vi "SubDiameter.vi"(7 "Calibration (1 pixel = ?um)":dbl=1.45, 8 "error in (no error)":errorcluster, 9 "Bot Wall":T1 {"Y" format="%.2f"; "X" format="%.2f"}, 10 "Top wall":T1 {"Y" format="%.2f"; "X" format="%.2f"}, 11 "AVI Path":path) -> (0 "error out":errorcluster, 1 "Y Mid":sgl[](array[numeric]), 2 "X Mid":sgl[](array[numeric]), 3 "Diameter":dbl[](array[numeric]))   [LabVIEW 2017]
uses:
  <vilib>/vision/NI_Vision_Development_Module.lvlib
panel:
  out "Vessel Diameter":dbl[](graph)
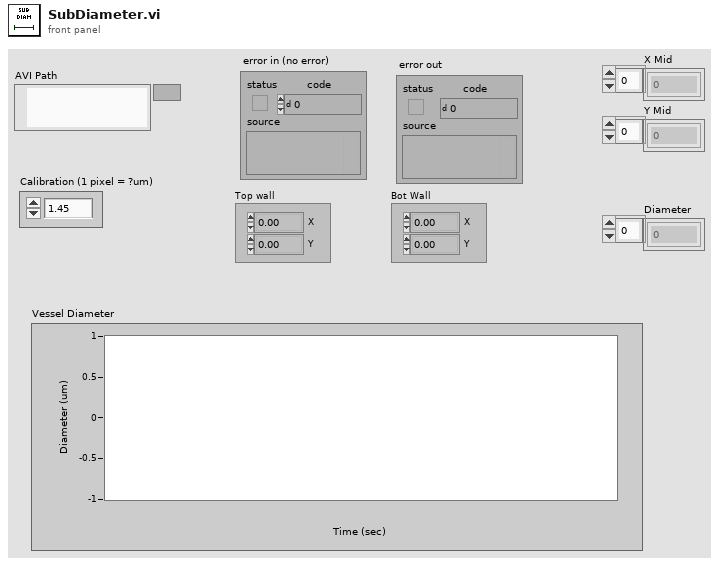
[diagram p1: front panel]
types:
  T1 = typedef "IMAQ Point" = cluster{"X":sgl, "Y":sgl}
  T2 = typedef "Image Type" = u32
  T3 = typedef "IMAQ AVI2 Refnum.ctl" = refnum<k20>
  T4 = cluster{"Width":u32, "Height":u32, "Frames Per Second":u32, "Codec":string, "Has Data":bool}
  T5 = typedef "IMAQ Image.ctl" = refnum<image>
  T6 = typedef "ROI Descriptor" = cluster{"Global Rectangle":i32[], "Contours":cluster{"ID":enum32{"External", "Internal"}, "Type":u32, "Coordinates":i32[]}[]}
  T7 = cluster{"Position":cluster{"x":sgl, "y":sgl}, "Angle":sgl, "Scale":sgl, "Score":sgl, "Bounding Box":cluster{"x":sgl, "y":sgl}[]}[]
  T8 = cluster{"Position":cluster{"x":sgl, "y":sgl}, "Position":cluster{"x":sgl, "y":sgl}}
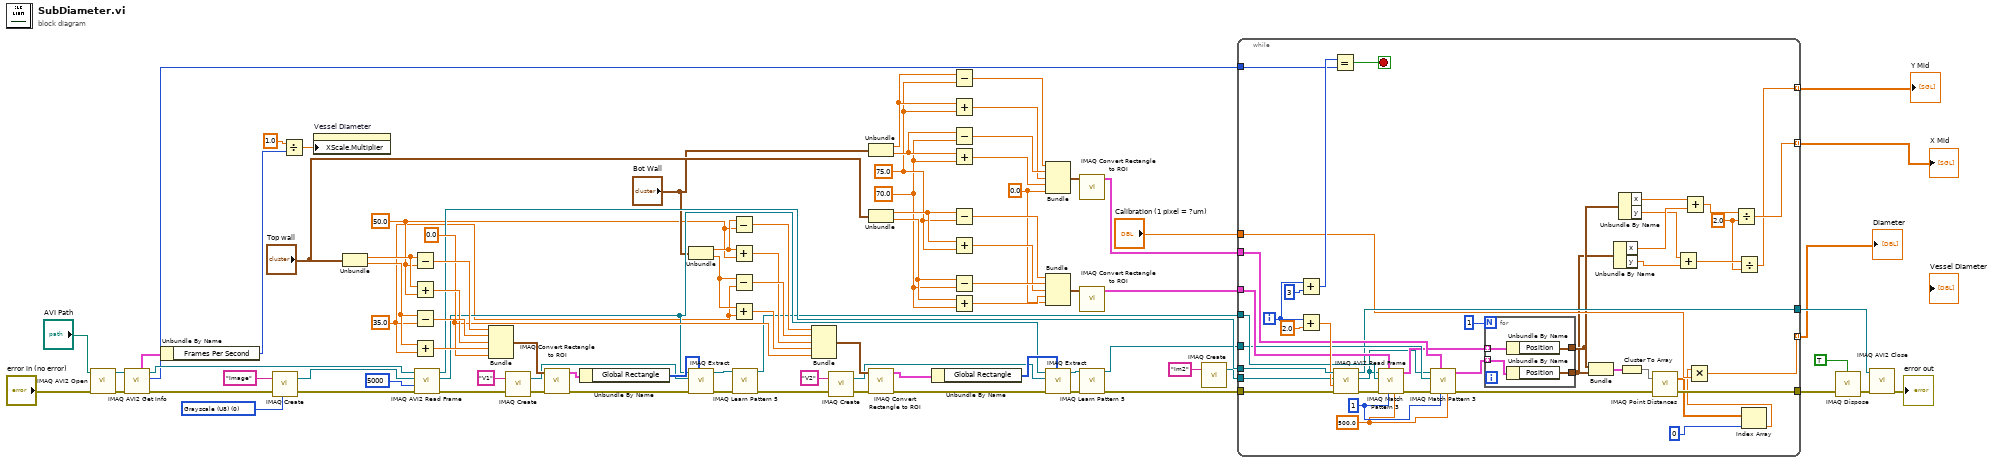
[diagram p0: block diagram]
diagram:
  w5 = 70.0 ("Search region offset (y)")
  w6 = 75.0 ("Search region offset (x)")
  w7 = 35.0 ("Reference offset (y)")
  w8 = 50.0 ("Reference offset (x)")
  w33 = 0.0
  w65 = 0.0
  w82 = T2 0 items=["Grayscale (U8)", "Grayscale (I16)", "Grayscale (SGL)", "Complex (CSG)", "RGB (U32)", "HSL (U32)", "RGB (U64)", "Grayscale (U16)"] ("Image Type")
  n1 = call "IMAQ AVI2 Open"("error in (no error)"="error in (no error)", "AVI File Path"="AVI Path") -> ("error out"=w88:errorcluster, "AVI Refnum"=w87:T3)  [unwired: 8 in]
  n2 = call "IMAQ AVI2 Get Info"("error in (no error)"=w88, "AVI Refnum"=w87) -> ("error out"=w85:errorcluster, "Number of Frames"=w46:u32, "AVI Refnum (duplicate)"=w80:T3, "Frame Data"=w23:T4)  [unwired: 5 in, 1 out]
  n3 = Unbundle By Name(w23) -> ("Frames Per Second"=w21:u32)
  n4 = call "IMAQ Create"("Image Name"="Image", "Image Type"=w82, "error in (no error)"=w85) -> ("New Image"=w84:T5, "error out"=w83:errorcluster)  [unwired: 2 in]
  n5 = Divide(x=1.0, y=w21) -> (x/y=w20:dbl)
  n6 = property on="Vessel Diameter" class="WFChart (strict)"("XScale.Multiplier"=w20) -> ()  [unwired: 2 in, 2 out]
  n7 = Unbundle("Top wall") -> ("X"=w79:sgl, "Y"=w78:sgl)
  n8 = Subtract(x=w79, y=w8) -> (x-y=w75:dbl)
  n9 = Add(x=w79, y=w8) -> (x+y=w73:dbl)
  n10 = Subtract(x=w78, y=w7) -> (x-y=w74:dbl)
  n11 = Add(x=w78, y=w7) -> (x+y=w72:dbl)
  n12 = call "IMAQ AVI2 Read Frame"("error in (no error)"=w83, "Frame Number"=u32 5000, "Image"=w84, "AVI Refnum"=w80) -> ("error out"=w11:errorcluster, "Image Out"=w52:T5, "AVI Refnum (duplicate)"=w47:T3)  [unwired: 5 in]
  n13 = Bundle(w75, w74, w73, w72, w65) -> (w71:cluster{dbl, dbl, dbl, dbl, dbl})  [unwired: 1 in]
  n14 = call "IMAQ Create"("Image Name"="V1", "error in (no error)"=w11) -> ("New Image"=w54:T5, "error out"=w62:errorcluster)  [unwired: 3 in]
  n15 = call "IMAQ Convert Rectangle to ROI"("error in (no error)"=w62, "Rectangle"=w71) -> ("error out"=w55:errorcluster, "ROI Descriptor"=w58:T6)  [unwired: 7 in]
  n16 = Unbundle By Name(w58) -> ("Global Rectangle"=w57:i32[])
  n17 = Unbundle("Bot Wall") -> ("X"=w77:sgl, "Y"=w76:sgl)
  n18 = call "IMAQ Extract"("Optional Rectangle"=w57, "error in (no error)"=w55, "Image Dst"=w54, "Image Src"=w52) -> ("error out"=w51:errorcluster, "Image Dst Out"=w50:T5)  [unwired: 6 in]
  n19 = Subtract(x=w77, y=w8) -> (x-y=w69:dbl)
  n20 = Add(x=w77, y=w8) -> (x+y=w67:dbl)
  n21 = Subtract(x=w76, y=w7) -> (x-y=w68:dbl)
  n22 = Add(x=w76, y=w7) -> (x+y=w66:dbl)
  n23 = call "IMAQ Learn Pattern 5"("Image"=w50, "error in (no error)"=w51) -> ("Template Image Out"=w30:T5, "error out"=w28:errorcluster)  [unwired: 11 in, 1 out]
  n24 = Bundle(w69, w68, w67, w66, w65) -> (w70:cluster{dbl, dbl, dbl, dbl, dbl})  [unwired: 1 in]
  n25 = call "IMAQ Create"("Image Name"="V2", "error in (no error)"=w28) -> ("New Image"=w53:T5, "error out"=w61:errorcluster)  [unwired: 3 in]
  n26 = Unbundle("Bot Wall") -> ("X"=w35:sgl, "Y"=w34:sgl)
  n27 = Unbundle("Top wall") -> ("X"=w41:sgl, "Y"=w40:sgl)
  n28 = call "IMAQ Convert Rectangle to ROI"("error in (no error)"=w61, "Rectangle"=w70) -> ("error out"=w56:errorcluster, "ROI Descriptor"=w60:T6)  [unwired: 7 in]
  n29 = Unbundle By Name(w60) -> ("Global Rectangle"=w59:i32[])
  n30 = Subtract(x=w35, y=w6) -> (x-y=w39:dbl)
  n31 = Add(x=w35, y=w6) -> (x+y=w37:dbl)
  n32 = Subtract(x=w34, y=w5) -> (x-y=w38:dbl)
  n33 = Add(x=w34, y=w5) -> (x+y=w36:dbl)
  n34 = Subtract(x=w41, y=w6) -> (x-y=w45:dbl)
  n35 = Add(x=w41, y=w6) -> (x+y=w43:dbl)
  n36 = Subtract(x=w40, y=w5) -> (x-y=w44:dbl)
  n37 = Add(x=w40, y=w5) -> (x+y=w42:dbl)
  n38 = Bundle(w39, w38, w37, w36, w33) -> (w25:cluster{dbl, dbl, dbl, dbl, dbl})  [unwired: 1 in]
  n39 = Bundle(w45, w44, w43, w42, w33) -> (w26:cluster{dbl, dbl, dbl, dbl, dbl})  [unwired: 1 in]
  n40 = call "IMAQ Extract"("Optional Rectangle"=w59, "error in (no error)"=w56, "Image Dst"=w53, "Image Src"=w52) -> ("error out"=w49:errorcluster, "Image Dst Out"=w48:T5)  [unwired: 6 in]
  n41 = call "IMAQ Convert Rectangle to ROI"("Rectangle"=w25) -> ("ROI Descriptor"=w31:T6)  [unwired: 8 in, 1 out]
  n42 = call "IMAQ Convert Rectangle to ROI"("Rectangle"=w26) -> ("ROI Descriptor"=w32:T6)  [unwired: 8 in, 1 out]
  n43 = call "IMAQ Learn Pattern 5"("Image"=w48, "error in (no error)"=w49) -> ("Template Image Out"=w29:T5, "error out"=w27:errorcluster)  [unwired: 11 in, 1 out]
  n44 = call "IMAQ Create"("Image Name"="Im2") -> ("New Image"=w18:T5)  [unwired: 4 in, 1 out]
  n45 = while {
    tunnel: w47 -> [w131]
    tunnel: w46 -> [w125]
    tunnel: w32 -> [w123]
    tunnel: w31 -> [w122]
    tunnel: w30 -> [w119]
    tunnel: w29 -> [w118]
    tunnel: w27 -> [w117]
    tunnel: [w109] -> w24
    tunnel: w18 -> [w107]
    tunnel: [w105] -> w15
    tunnel: "Calibration (1 pixel = ?um)" -> [w104]
    tunnel: [w103] -> w1 mode=indexing
    tunnel: [w93] -> w3 mode=indexing
    tunnel: [w92] -> w2 mode=indexing
    i -> [w128]
    stop <- w124 stop-if-true
    w94 = sgl 2.0 ("y")
    w108 = sgl 500.0 ("Minimum Match Score")
    w116 = 1 ("Number of Matches Requested")
    n46 = Add(x=w128, y=3) -> (x+y=w126:i32)
    n47 = Add(x=w128, y=2.0) -> (x+y=w129:dbl)
    n48 = Equal?(x=w126, y=w125) -> (x = y?=w124:bool)
    n49 = call "IMAQ AVI2 Read Frame"("error in (no error)"=w117, "Frame Number"=w129, "Image"=w107, "AVI Refnum"=w131) -> ("error out"=w121:errorcluster, "Image Out"=w112:T5, "AVI Refnum (duplicate)"=w109:T3)  [unwired: 5 in]
    n50 = call "IMAQ Match Pattern 3"("Minimum Match Score"=w108, "Number of Matches Requested"=w116, "ROI Descriptor"=w123, "error in (no error)"=w121, "Template Image"=w119, "Image"=w112) -> ("error out"=w120:errorcluster, "Matches"=w114:T7)  [unwired: 3 in, 1 out]
    n51 = call "IMAQ Match Pattern 3"("Minimum Match Score"=w108, "Number of Matches Requested"=w116, "ROI Descriptor"=w122, "error in (no error)"=w120, "Template Image"=w118, "Image"=w112) -> ("error out"=w106:errorcluster, "Matches"=w113:T7)  [unwired: 3 in, 1 out]
    n52 = for {
      N: 1 -> [_]
      tunnel: w114 -> [w135] mode=indexing
      tunnel: w113 -> [w134] mode=indexing
      tunnel: [w133] -> w102
      tunnel: [w132] -> w101
      n53 = Unbundle By Name(w135) -> ("Position"=w133:cluster{"x":sgl, "y":sgl})
      n54 = Unbundle By Name(w134) -> ("Position"=w132:cluster{"x":sgl, "y":sgl})
    }
    n55 = Bundle("Position"=w102, "Position"=w101) -> (w110:T8)  [unwired: 1 in]
    n56 = Unbundle By Name(w101) -> ("x"=w99:sgl, "y"=w96:sgl)
    n57 = Unbundle By Name(w102) -> ("x"=w100:sgl, "y"=w97:sgl)
    n58 = Cluster To Array(cluster=w110) -> (array=w111:cluster{"x":sgl, "y":sgl}[])
    n59 = call "IMAQ Point Distances"("Points"=w111, "error in (no error)"=w106) -> ("Distances"=w91:sgl[], "error out"=w105:errorcluster)  [unwired: 3 in]
    n60 = Add(x=w97, y=w96) -> (x+y=w95:sgl)
    n61 = Add(x=w100, y=w99) -> (x+y=w98:sgl)
    n62 = Divide(x=w98, y=w94) -> (x/y=w93:sgl)
    n63 = Divide(x=w95, y=w94) -> (x/y=w92:sgl)
    n64 = Index Array(array=w91, index=0 ("index (row)")) -> (element=w89:sgl)
    n65 = Multiply(x=w89, y=w104) -> (x*y=w103:dbl)
  }
  "Diameter" <- w1
  "X Mid" <- w3
  "Y Mid" <- w2
  n66 = call "IMAQ Dispose"("All Images? (No)"=TRUE, "error in (no error)"=w15) -> ("error out"=w17:errorcluster)  [unwired: 4 in]
  n67 = call "IMAQ AVI2 Close"("error in (no error)"=w17, "AVI Refnum"=w24) -> ("error out"=→"error out":errorcluster)  [unwired: 9 in]
